vi "Read Humidity.Slope.vi"(8 "error in (no error)":errorcluster, 11 "HTS221 in":refnum<class "HTS221.lvclass">) -> (0 "error out":errorcluster, 2 "Humidity.Slope":dbl, 3 "HTS221 out":refnum<class "HTS221.lvclass">)   [LabVIEW 2020, in "HTS221.lvclass"]
uses:
  HTS221.lvclass
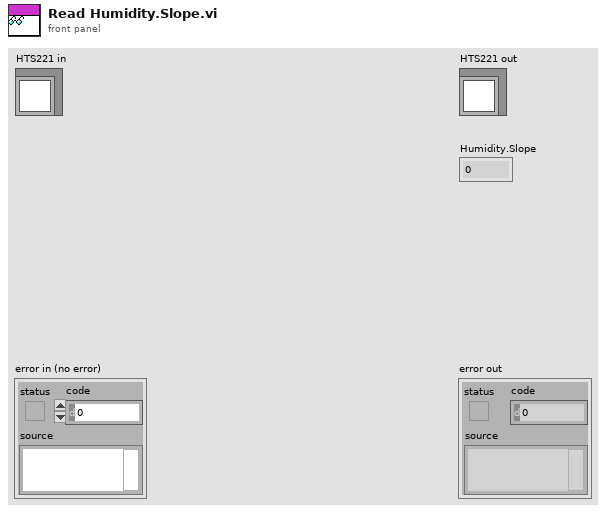
[diagram p1: front panel]
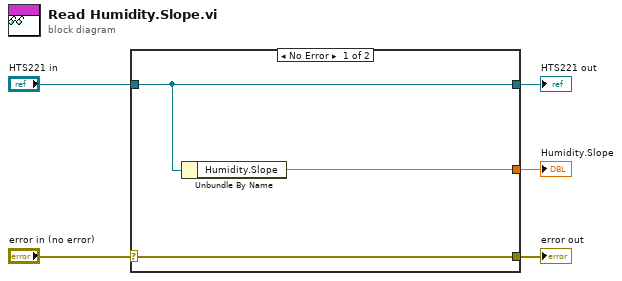
[diagram p0: block diagram]
diagram:
  n1 = case shown="No Error" "error in (no error)" {
    selector: "error in (no error)" -> [w8 w9]
    tunnel: [w8 w9] -> w4
    tunnel: [w7 w10] -> w2
    tunnel: "HTS221 in" -> [w7 w10]
    tunnel: [w6 _] -> w1
    frame No Error {
      n2 = Unbundle By Name(w7) -> ("Humidity.Slope"=w6:dbl)
    }
    frame Error {
    }
  }
  "error out" <- w4
  "HTS221 out" <- w2
  "Humidity.Slope" <- w1
